vi "Wago Reload PIDs.vi"(8 "Error In":errorcluster, 11 "Path":path) -> (0 "Error Out":errorcluster, 3 "Room PID Settings":T1 {"Room Dehumid Temperature I (*RM Dehum I1)" max=30000 step=1; "Room Dehumid Temperature P (*RM Dehum P1)" max=30000 step=1; "Room Cool Temperature I (*RM Cool I1)" max=30000 step=1; "Room Cool Temperature P (*RM Cool P1)" max=30000 step=1; "Room Heat I (*RM Heat I1)" max=30000 step=1; "Room Heat P (*RM Heat P1)" max=30000 step=1; "Room Humidity I (*RM Hum I1)" max=30000 step=1; "Room Humidity P (*RM Hum P1)" max=30000 step=1; "Room Dry I (*RM Dry I1)" max=30000 step=1; "Room Dry P(*RM Dry P1)" max=30000 step=1})   [LabVIEW 2016]
uses:
  Type Definitions/Wago Room PID Settings.ctl
  <vilib>/Utility/error.llb/whitespace.ctl
  <vilib>/Utility/file.llb/Read Delimited Spreadsheet (string).vi
panel:
  out "x*y 3":u16
  in  "x 2":u16
  in  "x":u16
  out "x*y 2":u16
  out "all rows":string[][](array[string])
  in  "File Name":string="RmPid8Stall.lup"
  out "appended path":path
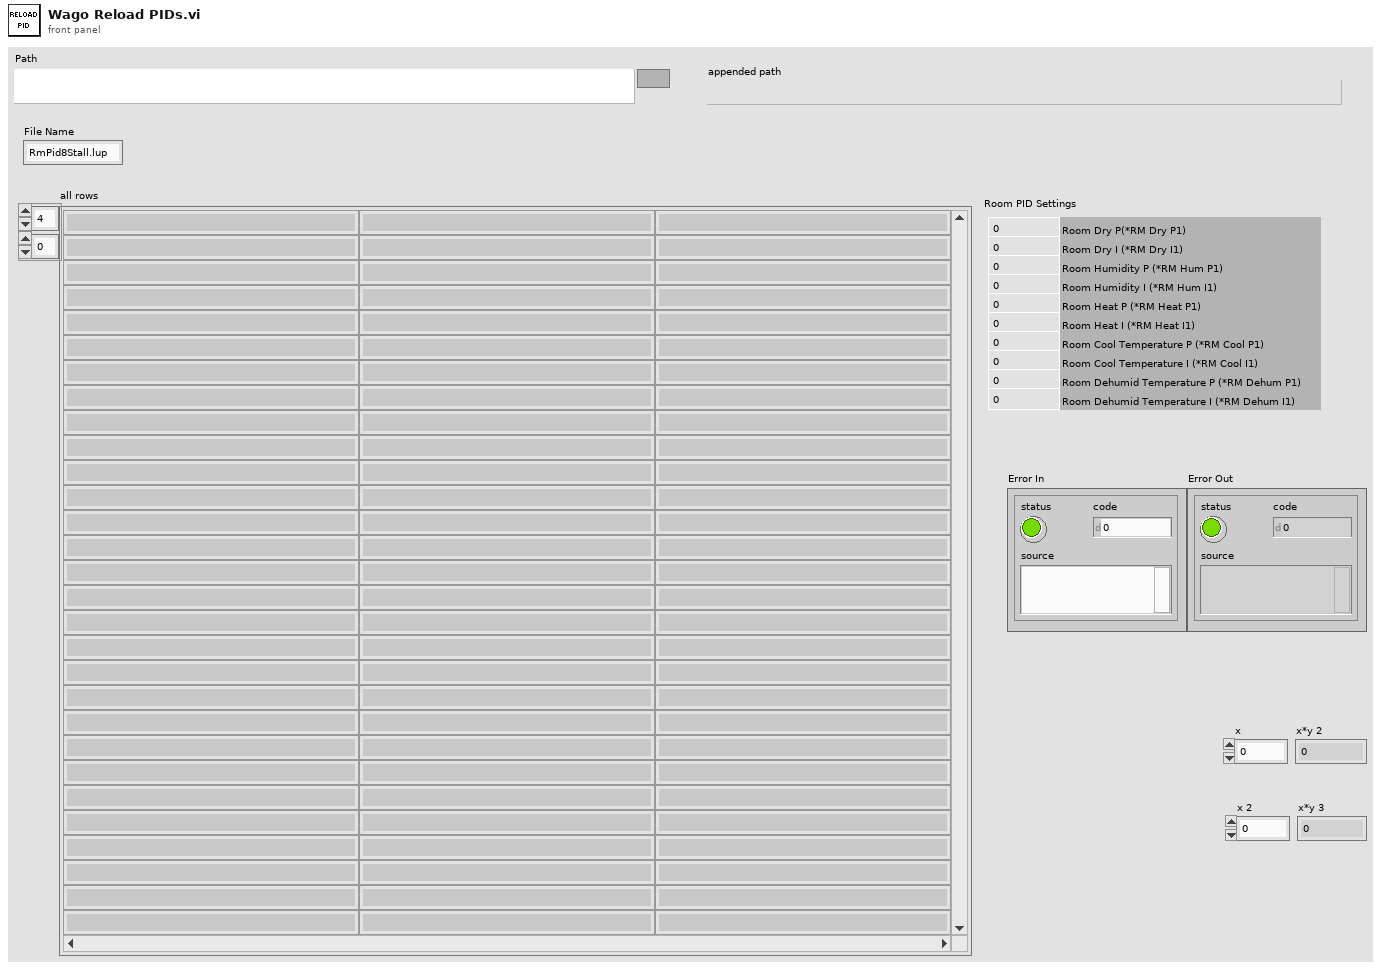
[diagram p1: front panel]
types:
  T1 = typedef "Wago Room PID Settings.ctl" = cluster{"Room Dry P(*RM Dry P1)":u16, "Room Dry I (*RM Dry I1)":u16, "Room Humidity P (*RM Hum P1)":u16, "Room Humidity I (*RM Hum I1)":u16, "Room Heat P (*RM Heat P1)":u16, "Room Heat I (*RM Heat I1)":u16, "Room Cool Temperature P (*RM Cool P1)":u16, "Room Cool Temperature I (*RM Cool I1)":u16, "Room Dehumid Temperature P (*RM Dehum P1)":u16, "Room Dehumid Temperature I (*RM Dehum I1)":u16}
  T2 = typedef "whitespace.ctl" = u16
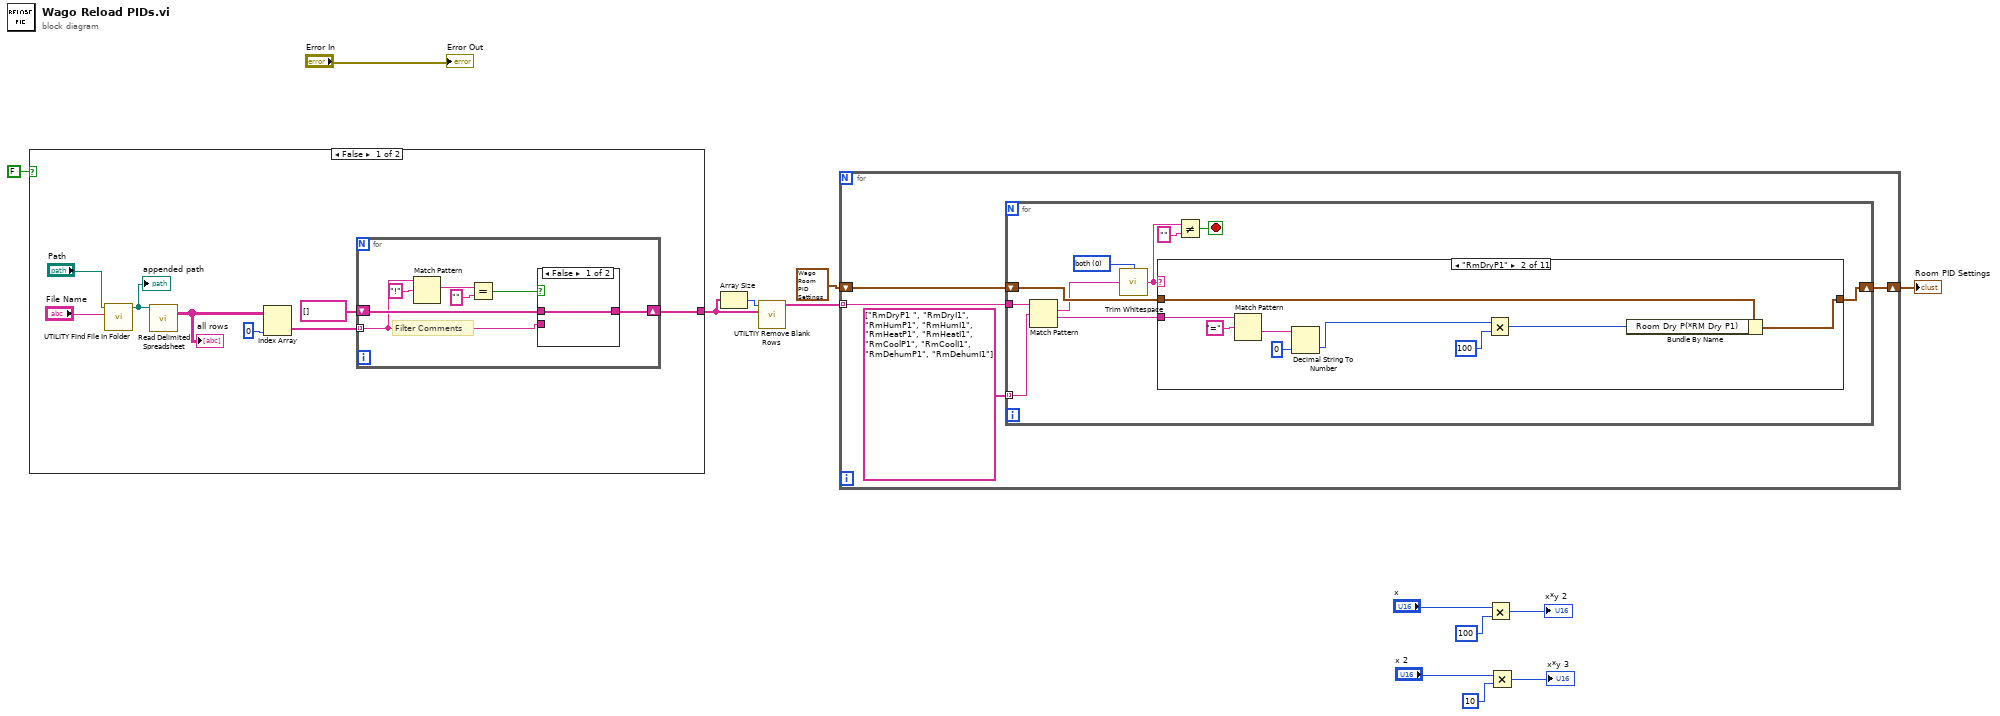
[diagram p0: block diagram]
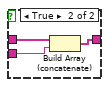
[diagram p2: hidden frame]
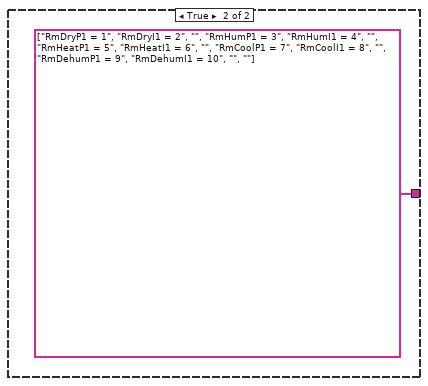
[diagram p3: hidden frame]
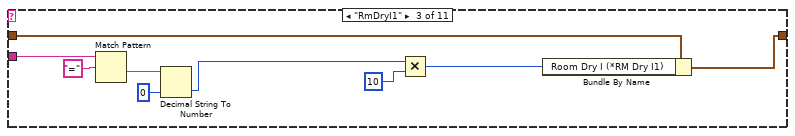
[diagram p5: hidden frame]
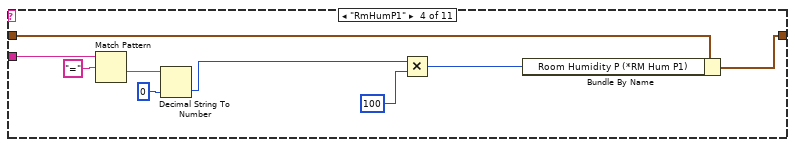
[diagram p6: hidden frame]
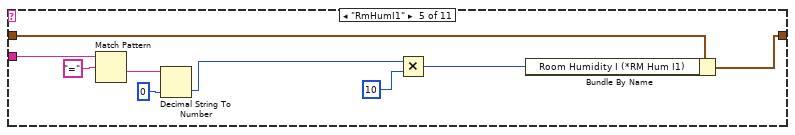
[diagram p7: hidden frame]
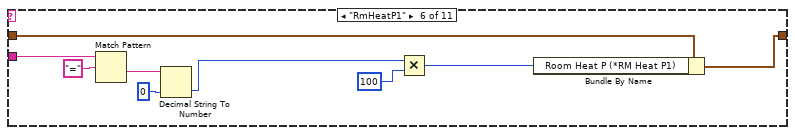
[diagram p8: hidden frame]
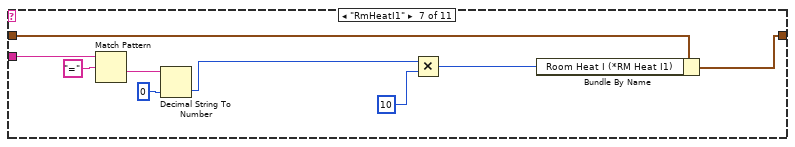
[diagram p9: hidden frame]
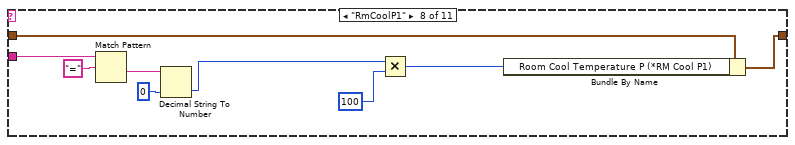
[diagram p10: hidden frame]
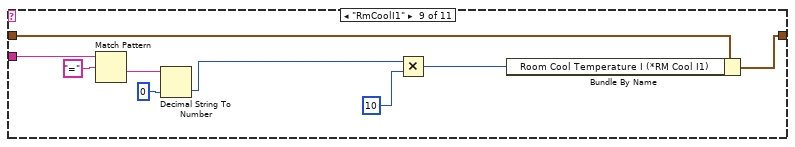
[diagram p11: hidden frame]
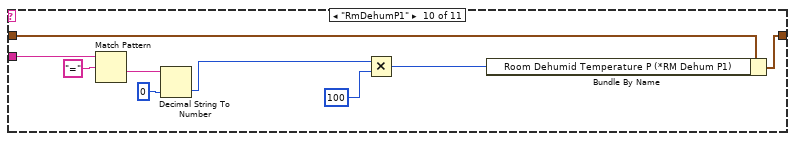
[diagram p12: hidden frame]
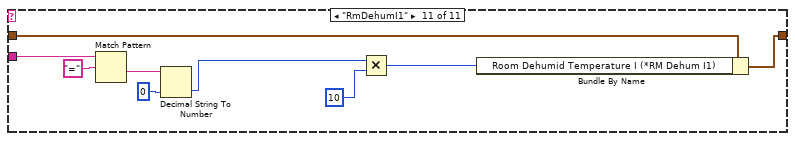
[diagram p13: hidden frame]
diagram:
  n1 = case shown="False" FALSE {
    tunnel: [w14 string[] ["RmDryP1 = 1", "RmDryI1 = 2", "", "RmHumP1 = 3", "RmHumI1 = 4", "", "RmHeatP1 = 5", "RmHeatI1 = 6", "", "RmCoolP1 = 7", "RmCoolI1 = 8", "", "RmDehumP1 = 9", "RmDehumI1 = 10", "", ""] ("Array 2")] -> w9
    frame False {
      n2 = call "UTILITY Find File In Folder.vi"("File Name"="File Name", "Path"="Path") -> ("appended path"=w19:path)  [unwired: 8 in, 1 out]
      "appended path" <- w19
      n3 = call-poly <vilib>:"Read Delimited Spreadsheet.vi"("file path (dialog if empty)"=w19) -> ("all rows"=w18:string[][])  [unwired: 9 in, 5 out]
      "all rows" <- w18
      n4 = Index Array(array=w18, index (col)=0 ("disabled index (col)")) -> (element=w17:string[])  [unwired: 1 in]
      n5 = for {
        tunnel: w17 -> [w22] mode=indexing
        shift-right: [w23] -> w14
        shift-left: string[] [] -> [w24]
        # "Filter Comments"
        n6 = Match Pattern(string=w22, regular expression="!") -> (match substring=w27:string)  [unwired: 1 in, 3 out]
        n7 = Equal?(x=w27, y="") -> (x = y?=w25:bool)
        n8 = case shown="False" w25 {
          tunnel: w24 -> [w29 w32]
          tunnel: [w29 w31] -> w23
          tunnel: w22 -> [_ w30]
          frame False {
          }
          frame True {
            n9 = Build Array (concatenate)(w32, w30) -> (w31:string[])
          }
        }
      }
    }
    frame True {
    }
  }
  n10 = Array Size(array=w9) -> (size(s)=w10:i32)
  n11 = call "UTILTIY Remove Blank Rows.vi"("all rows in"=w9, "Numeric"=w10) -> ("all rows out"=w8:string[])  [unwired: 9 in]
  n12 = for {
    tunnel: w8 -> [w35] mode=indexing
    shift-right: [w34] -> w12
    shift-left: T1 {"Room Dry P(*RM Dry P1)"=2, "Room Dry I (*RM Dry I1)"=1500, "Room Humidity P (*RM Hum P1)"=4, "Room Humidity I (*RM Hum I1)"=1500, "Room Heat P (*RM Heat P1)"=10, "Room Heat I (*RM Heat I1)"=200, "Room Cool Temperature P (*RM Cool P1)"=5, "Room Cool Temperature I (*RM Cool I1)"=600, "Room Dehumid Temperature P (*RM Dehum P1)"=5, "Room Dehumid Temperature I (*RM Dehum I1)"=600} ("Room PID Settings") -> [w37]
    n13 = for {
      tunnel: string[] ["RmDryP1 ", "RmDryI1", "RmHumP1", "RmHumI1", "RmHeatP1", "RmHeatI1", "RmCoolP1", "RmCoolI1", "RmDehumP1", "RmDehumI1"] -> [w44] mode=indexing
      tunnel: w35 -> [w43]
      shift-right: [w47] -> w34
      shift-left: w37 -> [w46]
      stop <- w41 stop-if-true
      w38 = T2 0 items=["both", "start of string", "end of string"] ("location (both)")
      n14 = Match Pattern(string=w43, regular expression=w44) -> (match substring=w40:string, after substring=w45:string)  [unwired: 1 in, 2 out]
      n15 = call <vilib>:"Trim Whitespace.vi"("string"=w40, "location (both)"=w38) -> ("trimmed string"=w39:string)
      n16 = case shown="\"RmDryP1\"" w39 {
        tunnel: w46 -> [w48 w57 w66 w74 w83 w92 w101 w110 w119 w128 w137]
        tunnel: [w48 w56 w65 w75 w84 w93 w102 w111 w120 w129 w138] -> w47
        tunnel: w45 -> [_ w52 w61 w70 w79 w88 w97 w106 w115 w124 w136]
        frame Default {
        }
        frame "RmDryP1" {
          n17 = Match Pattern(string=w52, regular expression="=") -> (after substring=w54:string)  [unwired: 1 in, 3 out]
          n18 = Decimal String To Number(string=w54, default (0L)=u16 0 ("default (0 I32)")) -> (number=w51:u16)  [unwired: 1 in, 1 out]
          n19 = Multiply(x=w51, y=u16 100) -> (x*y=w49:u16)
          n20 = Bundle By Name(cluster=w57, "Room Dry P(*RM Dry P1)"=w49) -> (w56:T1)
        }
        frame "RmDryI1" {
          n21 = Match Pattern(string=w61, regular expression="=") -> (after substring=w63:string)  [unwired: 1 in, 3 out]
          n22 = Decimal String To Number(string=w63, default (0L)=u16 0 ("default (0 I32)")) -> (number=w60:u16)  [unwired: 1 in, 1 out]
          n23 = Multiply(x=w60, y=u16 10) -> (x*y=w58:u16)
          n24 = Bundle By Name(cluster=w66, "Room Dry I (*RM Dry I1)"=w58) -> (w65:T1)
        }
        frame "RmHumP1" {
          n25 = Match Pattern(string=w70, regular expression="=") -> (after substring=w72:string)  [unwired: 1 in, 3 out]
          n26 = Decimal String To Number(string=w72, default (0L)=u16 0 ("default (0 I32)")) -> (number=w68:u16)  [unwired: 1 in, 1 out]
          n27 = Multiply(x=w68, y=u16 100) -> (x*y=w67:u16)
          n28 = Bundle By Name(cluster=w74, "Room Humidity P (*RM Hum P1)"=w67) -> (w75:T1)
        }
        frame "RmHumI1" {
          n29 = Match Pattern(string=w79, regular expression="=") -> (after substring=w81:string)  [unwired: 1 in, 3 out]
          n30 = Decimal String To Number(string=w81, default (0L)=u16 0 ("default (0 I32)")) -> (number=w77:u16)  [unwired: 1 in, 1 out]
          n31 = Multiply(x=w77, y=u16 10) -> (x*y=w76:u16)
          n32 = Bundle By Name(cluster=w83, "Room Humidity I (*RM Hum I1)"=w76) -> (w84:T1)
        }
        frame "RmHeatP1" {
          n33 = Match Pattern(string=w88, regular expression="=") -> (after substring=w90:string)  [unwired: 1 in, 3 out]
          n34 = Decimal String To Number(string=w90, default (0L)=u16 0 ("default (0 I32)")) -> (number=w86:u16)  [unwired: 1 in, 1 out]
          n35 = Multiply(x=w86, y=u16 100) -> (x*y=w85:u16)
          n36 = Bundle By Name(cluster=w92, "Room Heat P (*RM Heat P1)"=w85) -> (w93:T1)
        }
        frame "RmHeatI1" {
          n37 = Match Pattern(string=w97, regular expression="=") -> (after substring=w99:string)  [unwired: 1 in, 3 out]
          n38 = Decimal String To Number(string=w99, default (0L)=u16 0 ("default (0 I32)")) -> (number=w95:u16)  [unwired: 1 in, 1 out]
          n39 = Multiply(x=w95, y=u16 10) -> (x*y=w94:u16)
          n40 = Bundle By Name(cluster=w101, "Room Heat I (*RM Heat I1)"=w94) -> (w102:T1)
        }
        frame "RmCoolP1" {
          n41 = Match Pattern(string=w106, regular expression="=") -> (after substring=w108:string)  [unwired: 1 in, 3 out]
          n42 = Decimal String To Number(string=w108, default (0L)=u16 0 ("default (0 I32)")) -> (number=w104:u16)  [unwired: 1 in, 1 out]
          n43 = Multiply(x=w104, y=u16 100) -> (x*y=w103:u16)
          n44 = Bundle By Name(cluster=w110, "Room Cool Temperature P (*RM Cool P1)"=w103) -> (w111:T1)
        }
        frame "RmCoolI1" {
          n45 = Match Pattern(string=w115, regular expression="=") -> (after substring=w117:string)  [unwired: 1 in, 3 out]
          n46 = Decimal String To Number(string=w117, default (0L)=u16 0 ("default (0 I32)")) -> (number=w113:u16)  [unwired: 1 in, 1 out]
          n47 = Multiply(x=w113, y=u16 10) -> (x*y=w112:u16)
          n48 = Bundle By Name(cluster=w119, "Room Cool Temperature I (*RM Cool I1)"=w112) -> (w120:T1)
        }
        frame "RmDehumP1" {
          n49 = Match Pattern(string=w124, regular expression="=") -> (after substring=w126:string)  [unwired: 1 in, 3 out]
          n50 = Decimal String To Number(string=w126, default (0L)=u16 0 ("default (0 I32)")) -> (number=w122:u16)  [unwired: 1 in, 1 out]
          n51 = Multiply(x=w122, y=u16 100) -> (x*y=w121:u16)
          n52 = Bundle By Name(cluster=w128, "Room Dehumid Temperature P (*RM Dehum P1)"=w121) -> (w129:T1)
        }
        frame "RmDehumI1" {
          n53 = Match Pattern(string=w136, regular expression="=") -> (after substring=w134:string)  [unwired: 1 in, 3 out]
          n54 = Decimal String To Number(string=w134, default (0L)=u16 0 ("default (0 I32)")) -> (number=w131:u16)  [unwired: 1 in, 1 out]
          n55 = Multiply(x=w131, y=u16 10) -> (x*y=w130:u16)
          n56 = Bundle By Name(cluster=w137, "Room Dehumid Temperature I (*RM Dehum I1)"=w130) -> (w138:T1)
        }
      }
      n57 = Not Equal?(x=w39, y="") -> (x != y?=w41:bool)
    }
  }
  "Room PID Settings" <- w12
  n58 = Multiply(x="x", y=u16 100) -> (x*y=→"x*y 2":u16)
  n59 = Multiply(x="x 2", y=u16 10) -> (x*y=→"x*y 3":u16)
  "Error Out" <- "Error In"
